vi "curves.vi"() -> ()   [LabVIEW 2020]
panel:
  out "P CURVE":cluster{"V":dbl[], "I":dbl[]}(graph)
  out "I-V CURVE":cluster{"V":dbl[], "I":dbl[]}(graph)
  in  "I":dbl[](array[numeric])
  in  "V":dbl[](array[numeric])
  in  "stop":bool
  # "Maksimum Güç Noktasi izleyicili Fotovoltaik Sistemin                                                                            Labview Tabanli Kontrolü ve izlenmesi\n\n                  Doç.Dr. Ahmet Afsin KULAKSIZ\n                          Abdulkadir MÜHENDiS\n                                  KONYA - 2020"
  # "STC (1000 W/m2) / 37 C\nSenaryo - 2"
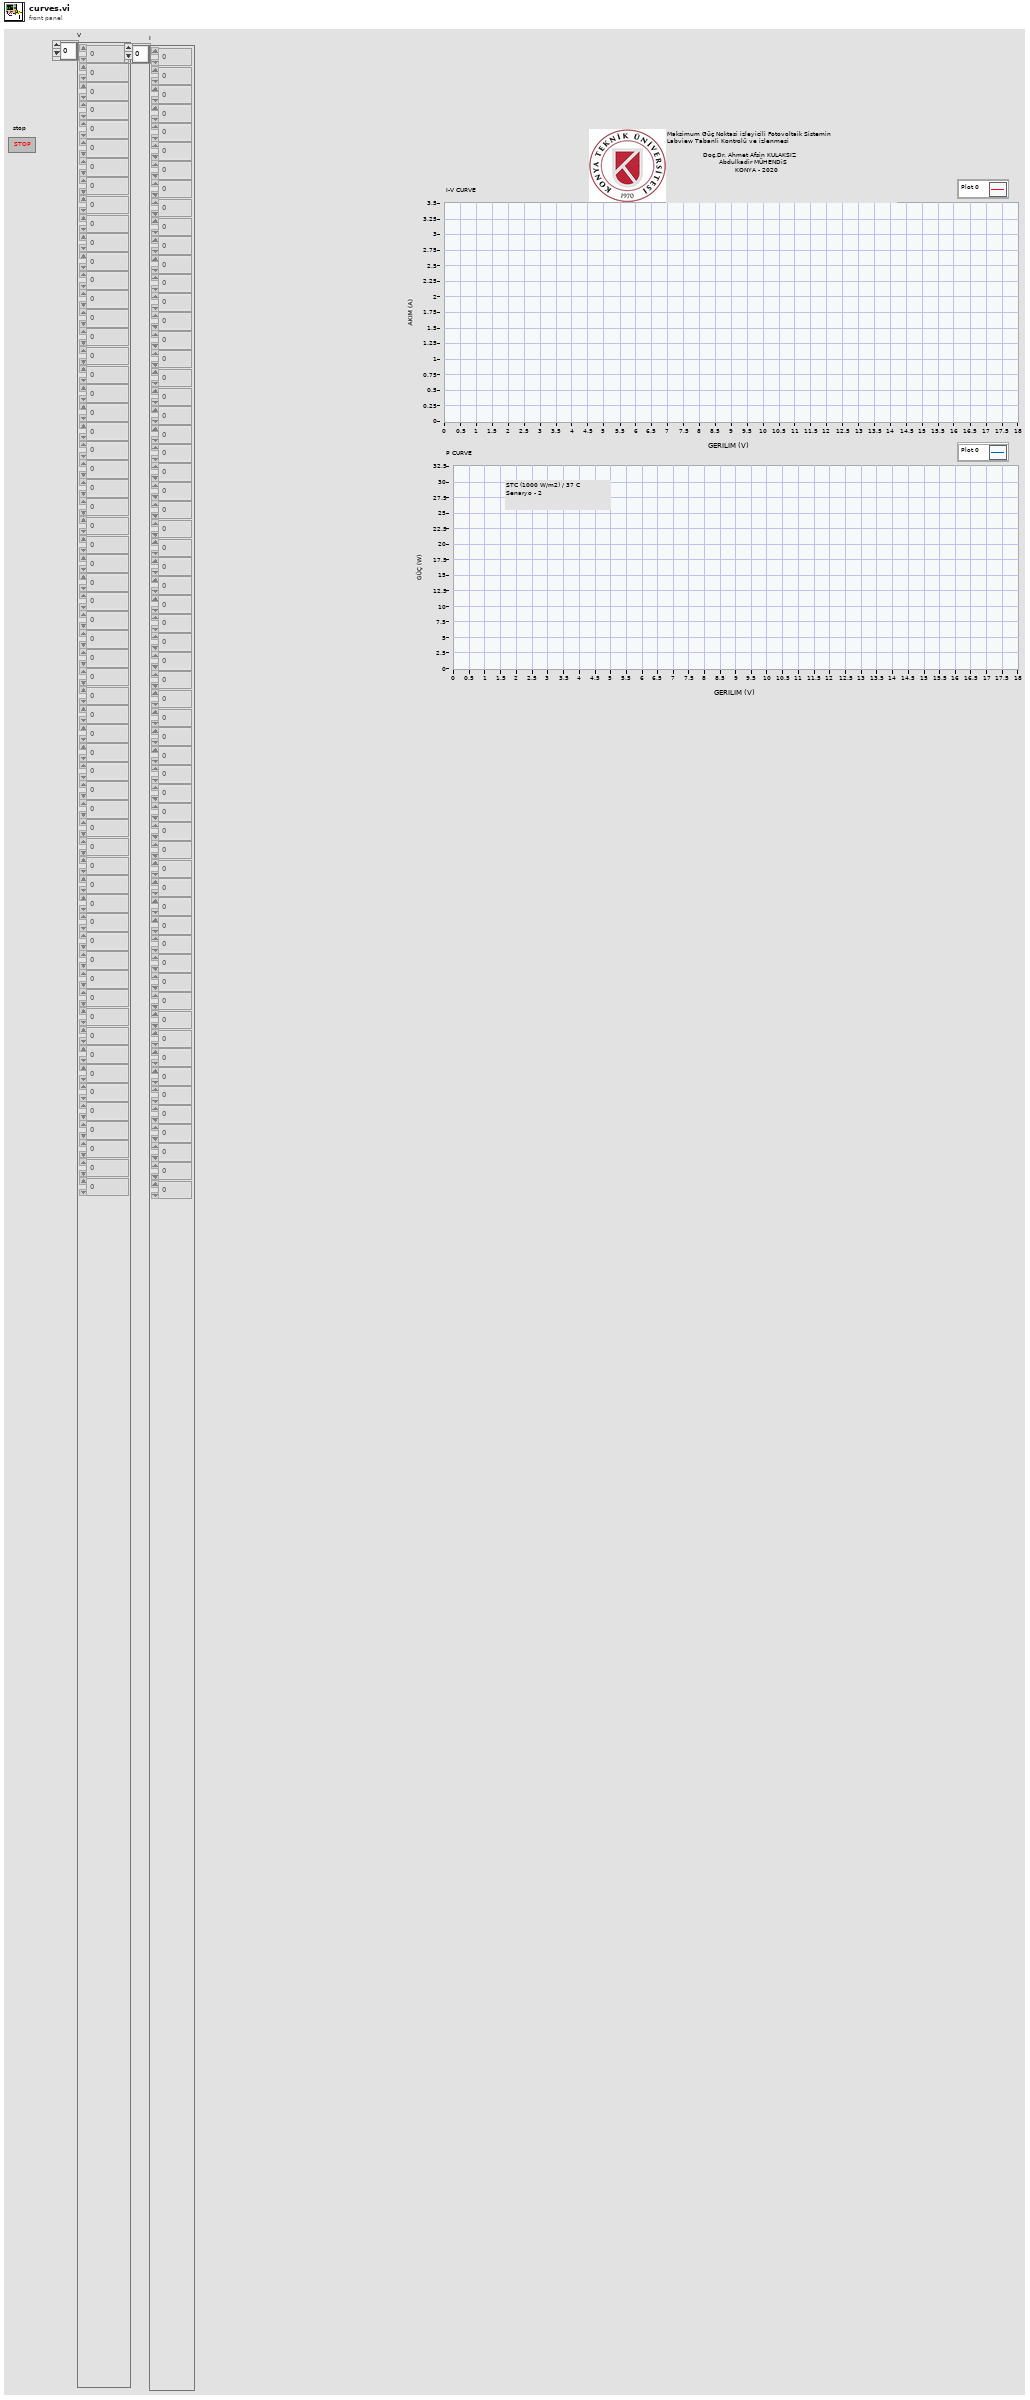
[diagram p1: front panel]
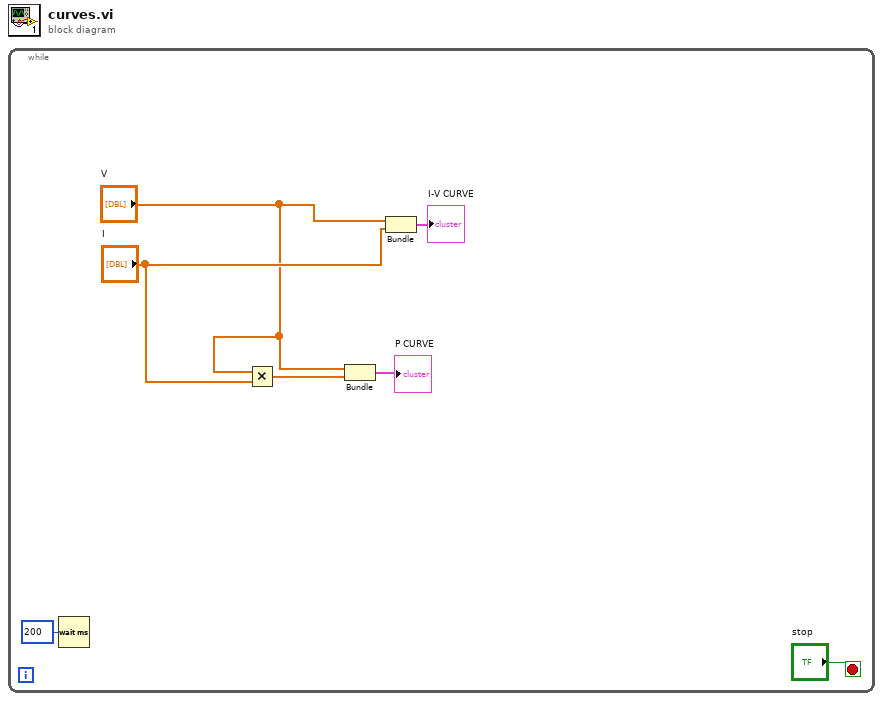
[diagram p0: block diagram]
diagram:
  n1 = while {
    stop <- "stop" stop-if-true
    n2 = Wait (ms)(milliseconds to wait=u32 200) -> ()  [unwired: 1 out]
    n3 = Multiply(x="V", y="I") -> (x*y=w3:dbl[])
    n4 = Bundle("V"="V", w3) -> (→"P CURVE":cluster{"V":dbl[], dbl[]})  [unwired: 1 in]
    n5 = Bundle("V"="V", "I"="I") -> (→"I-V CURVE":cluster{"V":dbl[], "I":dbl[]})  [unwired: 1 in]
  }
